vi "Set Message Window.vi"(11 "wnd":u32) -> (2 "function return":u32, 3 "wnd out":u32)   [LabVIEW 2018, in "AndorSDK.lvlib"]
doc: "EXPNETTYPE unsigned int WINAPI SetMessageWindow(HWND wnd);"
uses:
  AndorSDK.lvlib
  ATMCD32D.dll
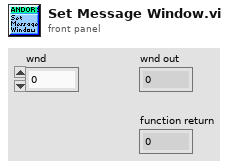
[diagram p1: front panel]
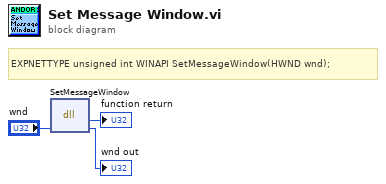
[diagram p0: block diagram]
diagram:
  # "EXPNETTYPE unsigned int WINAPI SetMessageWindow(HWND wnd);"
  n1 = dll-call lib="PTH2babs E\nPersönliches02 - Arbeit03-HiwijobsLabviewCodelibANDOR\tAndor SDK\nATMCD32D.*" fn="SetMessageWindow"("wnd"="wnd") -> (→"function return":u32, "wnd"=→"wnd out":u32)  [unwired: 3 in, 2 out]
